vi "TEST Blue to Green.vi"   [LabVIEW 2019]
uses:
  Global Var.vi
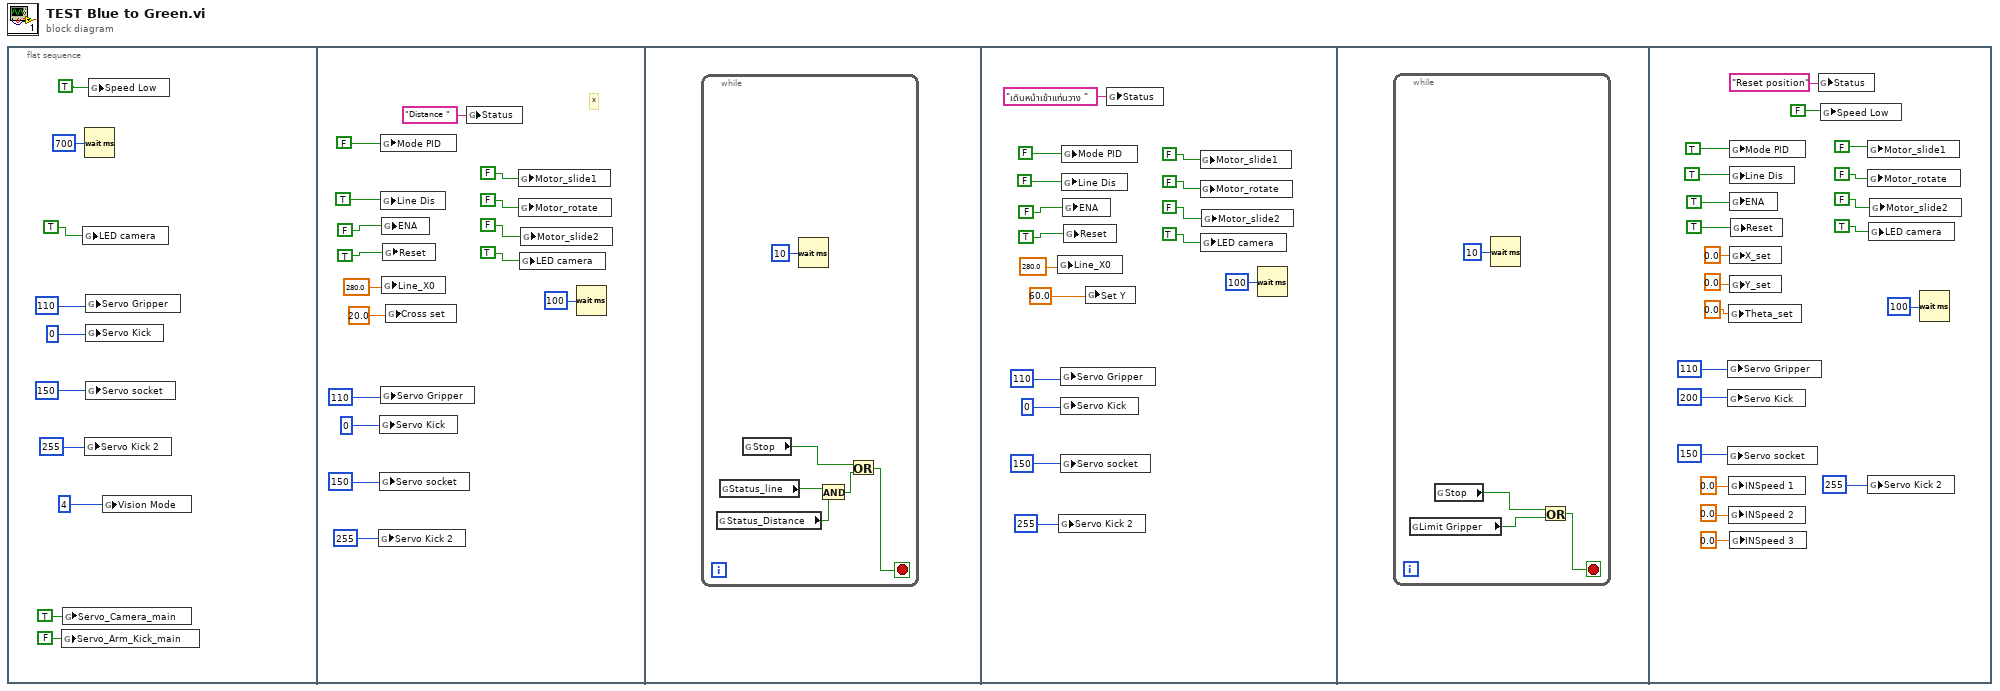
[diagram p0: block diagram]
diagram:
  n1 = flat-sequence {
    frame #0 {
      n2 = global write "Global Var.vi" "Servo_Arm_Kick_main"(FALSE ("Mode PID")) -> ()
      n3 = global write "Global Var.vi" "Servo_Camera_main"(TRUE ("Mode PID")) -> ()
      n4 = global write "Global Var.vi" "LED camera"(TRUE ("LED camera")) -> ()
      n5 = Wait (ms)(milliseconds to wait=u32 700) -> ()  [unwired: 1 out]
      n6 = global write "Global Var.vi" "Servo Kick 2"(u8 255 ("Servo Camera")) -> ()
      n7 = global write "Global Var.vi" "Servo Gripper"(u8 110 ("Servo Camera")) -> ()
      n8 = global write "Global Var.vi" "Servo Kick"(u8 0 ("Servo Camera")) -> ()
      n9 = global write "Global Var.vi" "Servo socket"(u8 150 ("Servo Camera")) -> ()
      n10 = global write "Global Var.vi" "Speed Low"(TRUE ("LED camera")) -> ()
      n11 = global write "Global Var.vi" "Vision Mode"(i16 4 ("Vision Mode")) -> ()
    }
    frame #1 {
      # "*"
      n12 = global write "Global Var.vi" "Servo Kick 2"(u8 255 ("Servo Camera")) -> ()
      n13 = global write "Global Var.vi" "Servo Kick"(u8 0 ("Servo Camera")) -> ()
      n14 = global write "Global Var.vi" "Servo socket"(u8 150 ("Servo Camera")) -> ()
      n15 = global write "Global Var.vi" "Mode PID"(FALSE ("Mode PID")) -> ()
      n16 = global write "Global Var.vi" "Line Dis"(TRUE ("Mode PID")) -> ()
      n17 = global write "Global Var.vi" "Servo Gripper"(u8 110 ("Servo Camera")) -> ()
      n18 = global write "Global Var.vi" "ENA"(FALSE ("ENA")) -> ()
      n19 = global write "Global Var.vi" "Line_X0"(280.0 ("Y_set")) -> ()
      n20 = global write "Global Var.vi" "Reset"(TRUE ("ENA")) -> ()
      n21 = global write "Global Var.vi" "Cross set"(20.0 ("Y_set")) -> ()
      n22 = global write "Global Var.vi" "Status"("Distance " ("Status")) -> ()
      n23 = global write "Global Var.vi" "Motor_slide1"(FALSE ("Mode PID")) -> ()
      n24 = global write "Global Var.vi" "Motor_rotate"(FALSE ("ENA")) -> ()
      n25 = global write "Global Var.vi" "LED camera"(TRUE ("LED camera")) -> ()
      n26 = global write "Global Var.vi" "Motor_slide2"(FALSE ("ENA")) -> ()
      n27 = Wait (ms)(milliseconds to wait=u32 100) -> ()  [unwired: 1 out]
    }
    frame #2 {
      n28 = while {
        stop <- w31 stop-if-true
        n29 = global read "Global Var.vi" "Status_Distance"() -> (w27:bool)
        n30 = global read "Global Var.vi" "Status_line"() -> (w28:bool)
        n31 = global read "Global Var.vi" "Stop"() -> (w30:bool)
        n32 = Wait (ms)(milliseconds to wait=u32 10) -> ()  [unwired: 1 out]
        n33 = And(x=w28, y=w27) -> (x .and. y?=w29:bool)
        n34 = Or(x=w30, y=w29) -> (x .or. y?=w31:bool)
      }
    }
    frame #3 {
      n35 = global write "Global Var.vi" "Line_X0"(280.0 ("Y_set")) -> ()
      n36 = global write "Global Var.vi" "Servo Kick 2"(u8 255 ("Servo Camera")) -> ()
      n37 = global write "Global Var.vi" "Servo Gripper"(u8 110 ("Servo Camera")) -> ()
      n38 = global write "Global Var.vi" "Servo Kick"(u8 0 ("Servo Camera")) -> ()
      n39 = global write "Global Var.vi" "Servo socket"(u8 150 ("Servo Camera")) -> ()
      n40 = global write "Global Var.vi" "Mode PID"(FALSE ("Mode PID")) -> ()
      n41 = global write "Global Var.vi" "Line Dis"(FALSE ("Mode PID")) -> ()
      n42 = global write "Global Var.vi" "ENA"(FALSE ("ENA")) -> ()
      n43 = global write "Global Var.vi" "Reset"(TRUE ("ENA")) -> ()
      n44 = global write "Global Var.vi" "Set Y"(60.0 ("Y_set")) -> ()
      n45 = global write "Global Var.vi" "Status"("เดินหน้าเข้าแท่นวาง " ("Status")) -> ()
      n46 = global write "Global Var.vi" "Motor_slide1"(FALSE ("Mode PID")) -> ()
      n47 = global write "Global Var.vi" "Motor_rotate"(FALSE ("ENA")) -> ()
      n48 = global write "Global Var.vi" "LED camera"(TRUE ("LED camera")) -> ()
      n49 = global write "Global Var.vi" "Motor_slide2"(FALSE ("ENA")) -> ()
      n50 = Wait (ms)(milliseconds to wait=u32 100) -> ()  [unwired: 1 out]
    }
    frame #4 {
      n51 = while {
        stop <- w51 stop-if-true
        n52 = global read "Global Var.vi" "Limit Gripper"() -> (w49:bool)
        n53 = global read "Global Var.vi" "Stop"() -> (w50:bool)
        n54 = Wait (ms)(milliseconds to wait=u32 10) -> ()  [unwired: 1 out]
        n55 = Or(x=w50, y=w49) -> (x .or. y?=w51:bool)
      }
    }
    frame #5 {
      n56 = global write "Global Var.vi" "Servo Gripper"(u8 110 ("Servo Camera")) -> ()
      n57 = global write "Global Var.vi" "Servo Kick"(u8 200 ("Servo Camera")) -> ()
      n58 = global write "Global Var.vi" "Servo socket"(u8 150 ("Servo Camera")) -> ()
      n59 = global write "Global Var.vi" "Theta_set"(0.0 ("Theta_set")) -> ()
      n60 = global write "Global Var.vi" "INSpeed 1"(0.0 ("X_set")) -> ()
      n61 = global write "Global Var.vi" "INSpeed 2"(0.0 ("Y_set")) -> ()
      n62 = global write "Global Var.vi" "Mode PID"(TRUE ("Mode PID")) -> ()
      n63 = global write "Global Var.vi" "Line Dis"(TRUE ("Mode PID")) -> ()
      n64 = global write "Global Var.vi" "ENA"(TRUE ("ENA")) -> ()
      n65 = global write "Global Var.vi" "X_set"(0.0 ("X_set")) -> ()
      n66 = global write "Global Var.vi" "Y_set"(0.0 ("Y_set")) -> ()
      n67 = global write "Global Var.vi" "INSpeed 3"(0.0 ("Theta_set")) -> ()
      n68 = global write "Global Var.vi" "Reset"(TRUE ("ENA")) -> ()
      n69 = global write "Global Var.vi" "Status"("Reset position" ("Status")) -> ()
      n70 = global write "Global Var.vi" "Speed Low"(FALSE ("LED camera")) -> ()
      n71 = global write "Global Var.vi" "Motor_slide1"(FALSE ("Mode PID")) -> ()
      n72 = global write "Global Var.vi" "Motor_rotate"(FALSE ("ENA")) -> ()
      n73 = global write "Global Var.vi" "Servo Kick 2"(u8 255 ("Servo Camera")) -> ()
      n74 = global write "Global Var.vi" "LED camera"(TRUE ("LED camera")) -> ()
      n75 = global write "Global Var.vi" "Motor_slide2"(FALSE ("ENA")) -> ()
      n76 = Wait (ms)(milliseconds to wait=u32 100) -> ()  [unwired: 1 out]
    }
  }
